vi "Connect.vi"(6 "Connect/Disconnect":bool, 8 "error in":errorcluster, 9 "Baud Rate":u32, 10 "ICommunicator Name":string, 11 "Interactor in":refnum<class "Interactor.lvclass">) -> (0 "error out":errorcluster, 3 "Interactor out":refnum<class "Interactor.lvclass">)   [LabVIEW 2024, in "Interactor.lvlib" / "Interactor.lvclass"]
uses:
  Interactor.lvclass
  Interactor.lvclass/Interactor.ctl
  Home Messages/CAN Adapter Connected Msg/CAN Adapter Connected Msg.lvclass
  CANopen Master/CANopen Master.lvclass
  HAL/Source/Instrument Manager/Instrument Manager.lvclass
  HAL/Source/Interfaces/ICommunicate/ICommunicate.lvclass
  HAL/Source/Config from JSON/Config from JSON.lvclass
  <vilib>/Utility/error.llb/DialogType.ctl
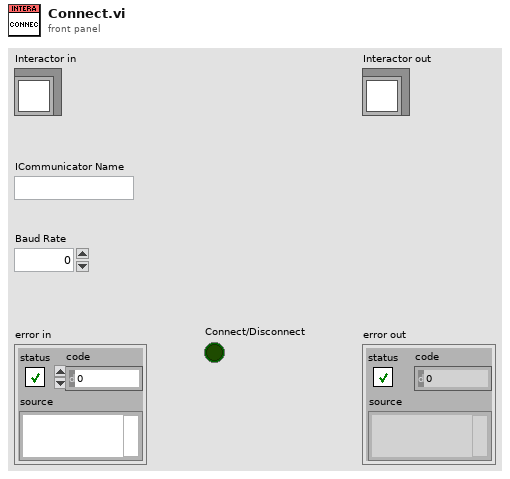
[diagram p1: front panel]
types:
  T1 = typedef "DialogType.ctl" = u16
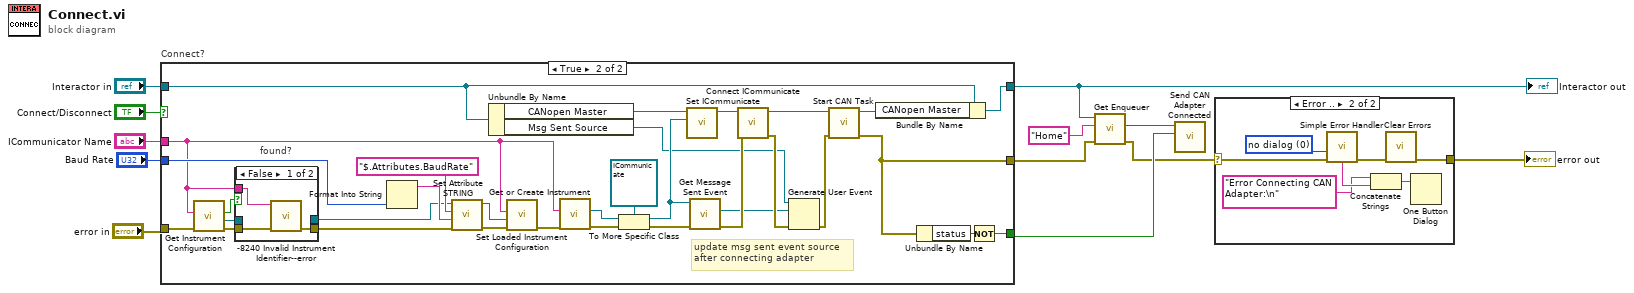
[diagram p0: block diagram]
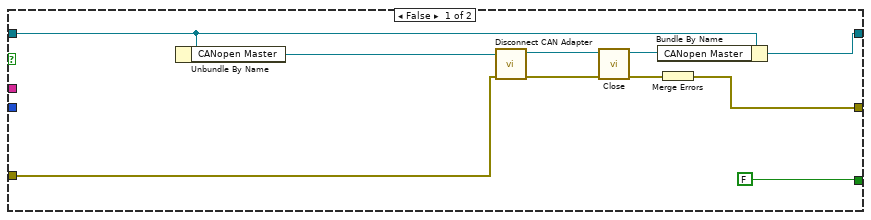
[diagram p2: hidden frame]
diagram:
  n1 = case "Connect?" shown="True" "Connect/Disconnect" {
    tunnel: "ICommunicator Name" -> [_ w32]
    tunnel: "error in" -> [w13 w45]
    tunnel: "Interactor in" -> [w20 w52]
    tunnel: [w14 w49] -> w6
    tunnel: [w16 w48] -> w3
    tunnel: [FALSE w53] -> w5
    tunnel: "Baud Rate" -> [_ w39]
    frame False {
      n2 = Unbundle By Name(w20) -> ("CANopen Master"=w22:refnum<class "CANopen Master.lvclass">)
      n3 = call-dynamic "Disconnect CAN Adapter.vi"("error in"=w13, "CANopen Master in"=w22) -> ("error out"=w19:errorcluster, "CANopen Master out"=w18:refnum<class "CANopen Master.lvclass">)  [unwired: 8 in]
      n4 = call "Close.vi"("error in"=w19, "CANopen Master in"=w18) -> ("error out"=w17:errorcluster, "CANopen Master out"=w15:refnum<class "CANopen Master.lvclass">)  [unwired: 8 in]
      n5 = Bundle By Name(cluster=w20, "CANopen Master"=w15) -> (w16:refnum<class "Interactor.lvclass">)
      n6 = Merge Errors(w17) -> (w14:errorcluster)
    }
    frame True {
      # "update msg sent event source\nafter connecting adapter"
      n7 = call "Get Instrument Configuration.vi"("Error In"=w45, "Instrument Identifier"=w32) -> ("Error Out"=w33:errorcluster, "Instrument Configuration"=w34:refnum<class "Config from JSON.lvclass">, "Found"=w35:bool)  [unwired: 7 in]
      n8 = case "found?" shown="False" w35 {
        tunnel: w34 -> [_ w58]
        tunnel: w33 -> [w57 w59]
        tunnel: w32 -> [w56 _]
        tunnel: [w55 w59] -> w31
        tunnel: [_ w58] -> w30
        frame False {
          n9 = call "-8240 Invalid Instrument Identifier--error.vi"("error in"=w57, "Instrument Identifier"=w56) -> ("error out"=w55:errorcluster)  [unwired: 9 in]
        }
        frame True {
        }
      }
      n10 = Format Into String(w39) -> (resulting string=w38:string)  [unwired: 3 in, 1 out]
      n11 = call-dynamic "Set Attribute STRING.vi"("error in"=w31, "Value"=w38, "Path"="$.Attributes.BaudRate", "Config from JSON in"=w30) -> ("error out"=w37:errorcluster, "Config from JSON out"=w36:refnum<class "Config from JSON.lvclass">)  [unwired: 6 in]
      n12 = Unbundle By Name(w52) -> ("CANopen Master"=w51:refnum<class "CANopen Master.lvclass">, "Msg Sent Source"=w23:refnum<user-event>)
      n13 = call "Set Loaded Instrument Configuration.vi"("Error In"=w37, "Config from JSON"=w36, "Instrument Identifier"=w32) -> ("Error Out"=w44:errorcluster)  [unwired: 8 in]
      n14 = call "Get or Create Instrument.vi"("Error In"=w44, "Instrument Identifier"=w32) -> ("Error Out"=w43:errorcluster, "IInstrument"=w42:refnum<class "IInstrument.lvclass">)  [unwired: 8 in]
      n15 = To More Specific Class(target class=refnum<class "ICommunicate.lvclass"> refnum ("ICommunicate.lvclass"), reference=w42, error in=w43) -> (specific class reference=w28:refnum<class "ICommunicate.lvclass">, error out=w29:errorcluster)
      n16 = call "Set ICommunicate.vi"("ICommunicate"=w28, "CANopen Master in"=w51) -> ("CANopen Master out"=w47:refnum<class "CANopen Master.lvclass">)  [unwired: 9 in]
      n17 = call-dynamic "Get Message Sent Event.vi"("error in"=w29, "ICommunicate in"=w28) -> ("error out"=w27:errorcluster, "Msg Sent Event"=w24:refnum<user-event>)  [unwired: 7 in, 1 out]
      n18 = call "Connect ICommunicate.vi"("error in (no error)"=w27, "CANopen Master in"=w47) -> ("error out"=w26:errorcluster, "CANopen Master out"=w46:refnum<class "CANopen Master.lvclass">)  [unwired: 8 in]
      n19 = Generate User Event(user event=w23, event data cluster=w24, error in=w26) -> (error out=w25:errorcluster)  [unwired: 1 in, 1 out]
      n20 = call "Start CAN Task.vi"("error in"=w25, "CANopen Master in"=w46) -> ("error out"=w49:errorcluster, "CANopen Master out"=w50:refnum<class "CANopen Master.lvclass">)  [unwired: 8 in]
      n21 = Bundle By Name(cluster=w52, "CANopen Master"=w50) -> (w48:refnum<class "Interactor.lvclass">)
      n22 = Unbundle By Name(w49) -> ("status"=w54:bool)
      n23 = Not(x=w54) -> (.not. x?=w53:bool)
    }
  }
  "Interactor out" <- w3
  n24 = call "Get Enqueuer.vi"("error in"=w6, "Ident"="Home", "Interactor in"=w3) -> ("error out"=w4:errorcluster, "Enq"=w8:refnum<class "Message Enqueuer.lvclass">)  [unwired: 6 in, 1 out]
  n25 = call "Send CAN Adapter Connected.vi"("CAN Adapter Connected?"=w5, "Message Enqueuer"=w8) -> ()  [unwired: 8 in, 2 out]
  n26 = case shown="Error .." w4 {
    selector: w4 -> [w60 w67]
    tunnel: [w60 w61] -> w1
    frame No Error {
    }
    frame Error {
      w65 = T1 0 items=["no dialog", "OK message", "continue or stop message", "OK message + warnings", "continue/stop + warnings"] ("type of dialog (OK msg:1)")
      n27 = call <vilib>:"Simple Error Handler.vi"("type of dialog (OK msg:1)"=w65, "error in (no error)"=w67) -> ("error out"=w66:errorcluster, "message"=w63:string)  [unwired: 3 in, 3 out]
      n28 = Concatenate Strings("Error Connecting CAN Adapter:\n" ("string"), w63) -> (w64:string)
      n29 = call <vilib>:"Clear Errors.vi"("error in (no error)"=w66) -> ("error out"=w61:errorcluster)  [unwired: 5 in, 1 out]
      n30 = One Button Dialog(message=w64) -> ()  [unwired: 1 in, 1 out]
    }
  }
  "error out" <- w1
